vi "niRFUtil WFM Moving Average (complex array).vi"(0 "Array In":T1 format="%.2f", 5 "Averaging Window (samples)":i32=20) -> (4 "Averaged Array Out":T1 format="%.2f")   [LabVIEW 2015, in "niRFUtil.lvlib"]
uses:
  niRFUtil.lvlib
  Includes/niRFUtil INC Complex Array.ctl
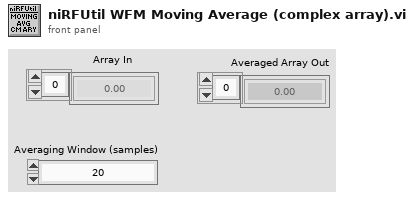
[diagram p1: front panel]
types:
  T1 = typedef "niRFUtil.lvlib/niRFUtil INC Complex Array.ctl" = csg[]
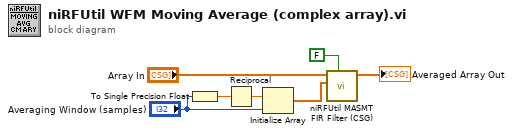
[diagram p0: block diagram]
diagram:
  n1 = To Single Precision Float(number="Averaging Window (samples)") -> (single precision float=w7:sgl)
  n2 = Reciprocal(x=w7) -> (1/x=w6:sgl)
  n3 = Initialize Array(w6, "Averaging Window (samples)") -> (w3:sgl[])
  n4 = call "niRFUtil MASMT FIR Filter (CSG).vi"("continue?"=FALSE, "FIR Coefficients"=w3, "X"="Array In") -> ("Filtered X"=→"Averaged Array Out":csg[])  [unwired: 7 in, 1 out]
